vi "editGraphData.vi"(8 "error in (no error)":errorcluster, 10 "Data 2":T1[](array[typedef]), 11 "Data":T1[](array[typedef])) -> (0 "error out":errorcluster, 3 "Data 3":T1[](array[typedef]))   [LabVIEW 2020]
uses:
  <vilib>/Stadlmann TEC/OXYGEN Datastream/VIs/Data Aquasation/TypeDefs/DataPoint_Double.ctl
  <vilib>/Stadlmann TEC/OXYGEN Datastream/OXYGEN_Datastream.lvlib
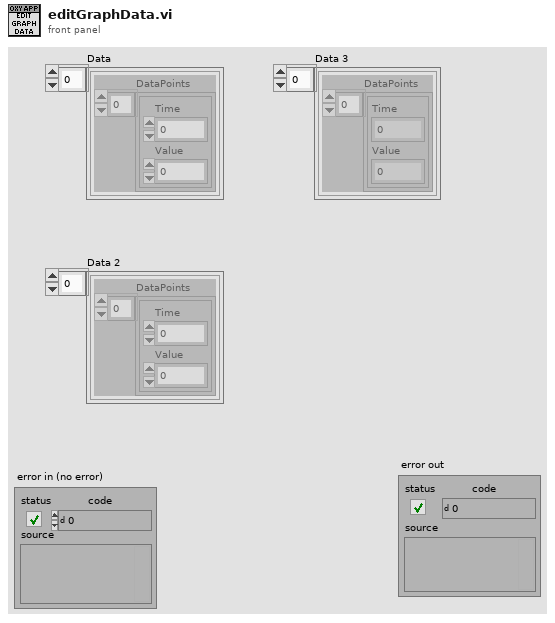
[diagram p1: front panel]
types:
  T1 = typedef "OXYGEN_Datastream.lvlib/DataPoint_Double.ctl" = cluster{"DataPoints":cluster{"Time":dbl, "Value":dbl}[]}
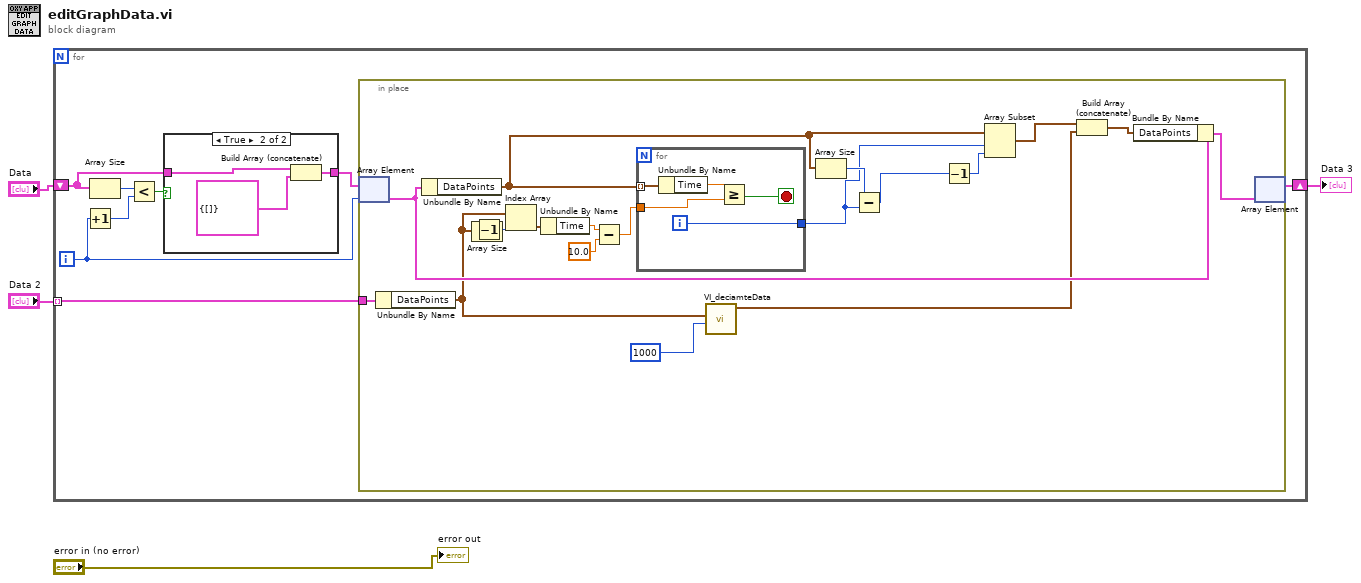
[diagram p0: block diagram]
diagram:
  n1 = for {
    shift-right: [w5] -> w1
    shift-left: "Data" -> [w9]
    tunnel: "Data 2" -> [w8] mode=indexing
    i -> [w7]
    n2 = Increment(x=w7) -> (x+1=w11:i32)
    n3 = Array Size(array=w9) -> (size(s)=w12:i32)
    n4 = Less?(x=w12, y=w11) -> (x < y?=w10:bool)
    n5 = case shown="True" w10 {
      tunnel: w9 -> [w37 w40]
      tunnel: [w37 w38] -> w6
      frame False {
      }
      frame True {
        n6 = Build Array (concatenate)(w40, T1 {"DataPoints"=[]} ("Data")) -> (w38:T1[])
      }
    }
    n7 = in-place {
      in-place-border: w8 -> [w31]
      n8 = in-place-array #1(w6, w7) -> (w27:T1)
      n9 = Unbundle By Name(w31) -> ("DataPoints"=w13:cluster{"Time":dbl, "Value":dbl}[])
      n10 = Unbundle By Name(w27) -> ("DataPoints"=w22:cluster{"Time":dbl, "Value":dbl}[])
      n11 = Array Size(array=w13) -> (size(s)=w15:i32)
      n12 = Decrement(x=w15) -> (x-1=w17:i32)
      n13 = Index Array(array=w13, index=w17) -> (element=w21:cluster{"Time":dbl, "Value":dbl})
      n14 = Unbundle By Name(w21) -> ("Time"=w20:dbl)
      n15 = Subtract(x=w20, y=10.0) -> (x-y=w18:dbl)
      n16 = for {
        tunnel: w22 -> [w34] mode=indexing
        tunnel: w18 -> [w35]
        tunnel: [w33] -> w25
        i -> [w33]
        stop <- w32 stop-if-true
        n17 = Unbundle By Name(w34) -> ("Time"=w36:dbl)
        n18 = Greater Or Equal?(x=w36, y=w35) -> (x >= y?=w32:bool)
      }
      n19 = call "VI_deciamteData.vi"("Factor"=1000 ("y"), "DataPoints"=w13) -> ("Array"=w16:cluster{"Time":dbl, "Value":dbl}[])  [unwired: 9 in]
      n20 = Array Size(array=w22) -> (size(s)=w28:i32)
      n21 = Subtract(x=w28, y=w25) -> (x-y=w24:i32)
      n22 = Decrement(x=w24) -> (x-1=w23:i32)
      n23 = Array Subset(array=w22, index=w25, length=w23) -> (w29:cluster{"Time":dbl, "Value":dbl}[])
      n24 = Build Array (concatenate)(w29, w16) -> (w30:cluster{"Time":dbl, "Value":dbl}[])
      n25 = Bundle By Name(cluster=w27, "DataPoints"=w30) -> (w26:T1)
      n26 = in-place-array #1(w26) -> (w5:T1[])  [unwired: 1 out]
    }
  }
  "Data 3" <- w1
  "error out" <- "error in (no error)"
